vi "Get Bit.vi"(0 "OWEN HMI in":refnum<class "OWEN HMI.lvclass">, 7 "bit":T1, 11 "error in (no error)":errorcluster) -> (4 "OWEN HMI out":refnum<class "OWEN HMI.lvclass">, 6 "value":bool, 15 "error out":errorcluster)   [LabVIEW 2019, in "OWEN HMI.lvclass"]
uses:
  OWEN HMI.lvclass
  Bit.ctl
  OWEN HMI.lvclass/OWEN HMI.ctl
  Words.ctl
  0a1eb2bf-41e0-46d0-9208-a62996f842b1.vi
  <vilib>/NI/Modbus Library/API/Master/Modbus Master.lvclass
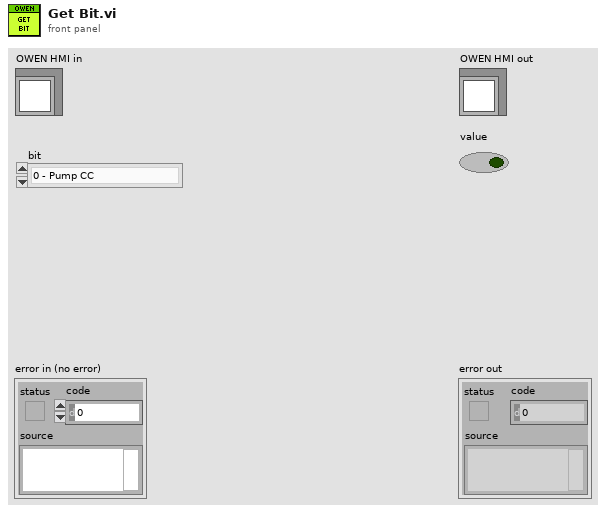
[diagram p1: front panel]
types:
  T1 = typedef "OWEN HMI.lvclass/Bit.ctl" = enum16{"0 - Pump CC", "1 - Pump SO", "2 - Alarm", "3 - Warning", "4 - DUT", "5 - CHMBR"}
  T2 = typedef "OWEN HMI.lvclass/Words.ctl" = enum16{"0 - Bits", "1 - Level CC", "2 - Temp CC", "3 - Level SO", "4 - Temp SO"}
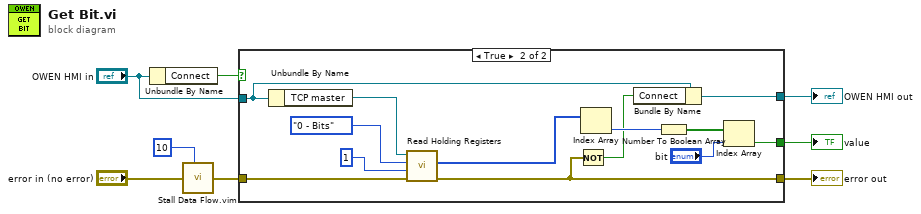
[diagram p0: block diagram]
diagram:
  n1 = Unbundle By Name("OWEN HMI in") -> ("Connect"=w6:bool)
  n2 = call "Stall Data Flow.vim"("value in"="error in (no error)", "milliseconds to wait"=u32 10) -> ("value out"=w1:errorcluster)  [unwired: 1 out]
  n3 = case shown="True" w6 {
    tunnel: w1 -> [w10 w23]
    tunnel: [_ w18] -> w8
    tunnel: [w10 w12] -> w7
    tunnel: [w9 w13] -> w4
    tunnel: "OWEN HMI in" -> [w9 w14]
    frame False {
    }
    frame True {
      n4 = Unbundle By Name(w14) -> ("TCP master"=w22:refnum<class "Modbus Master.lvclass">)
      n5 = call-dynamic "Read Holding Registers.vi"("error in"=w23, "number of inputs"=u16 1, "starting address"=Words."0 - Bits" ("Word"), "Modbus master in"=w22) -> ("error out"=w12:errorcluster, "register values"=w21:u16[])  [unwired: 5 in, 1 out]
      n6 = Not(x=w12) -> (.not. x?=w11:bool)
      n7 = Index Array(array=w21) -> (element=w20:u16)  [unwired: 1 in]
      n8 = Bundle By Name(cluster=w14, "Connect"=w11) -> (w13:refnum<class "OWEN HMI.lvclass">)
      n9 = Number To Boolean Array(number=w20) -> (Boolean array=w19:bool[])
      n10 = Index Array(array=w19, index="bit") -> (element=w18:bool)
    }
  }
  "error out" <- w7
  "OWEN HMI out" <- w4
  "value" <- w8
